vi "LidarLiteV3_I2C_Sample.vi"() -> ()   [LabVIEW 2019]
uses:
  <vilib>/ptbypt/NI_PtbyPt.lvlib
  <vilib>/Rock Robotics/SystemInterfaces/i2clib/i2c_bus.ctl
panel:
  out "Signal Stength":dbl format="%14.0f"
  in  "I2C Bus":T1
  in  "Average FIlter\nSamples":i32=5
  in  "Calibration\nOffset":dbl format="%#_13g"
  in  "Calibration \nGain":dbl=1.0 format="%#_13g"
  out "Lidar Distance Chart":cluster{dbl, "mean":dbl, dbl}(graph)
  out "Distance\nAverage FIlter\nFeet":dbl format="%19.3f"
  out "Distance\nFeet":dbl format="%19.3f"
  # "Read Lidar Lite V3 Using I2C Communications"
  # "Set these values before\nexecuting program"
  # "These values can be\nchanged while the \nprogram is running"
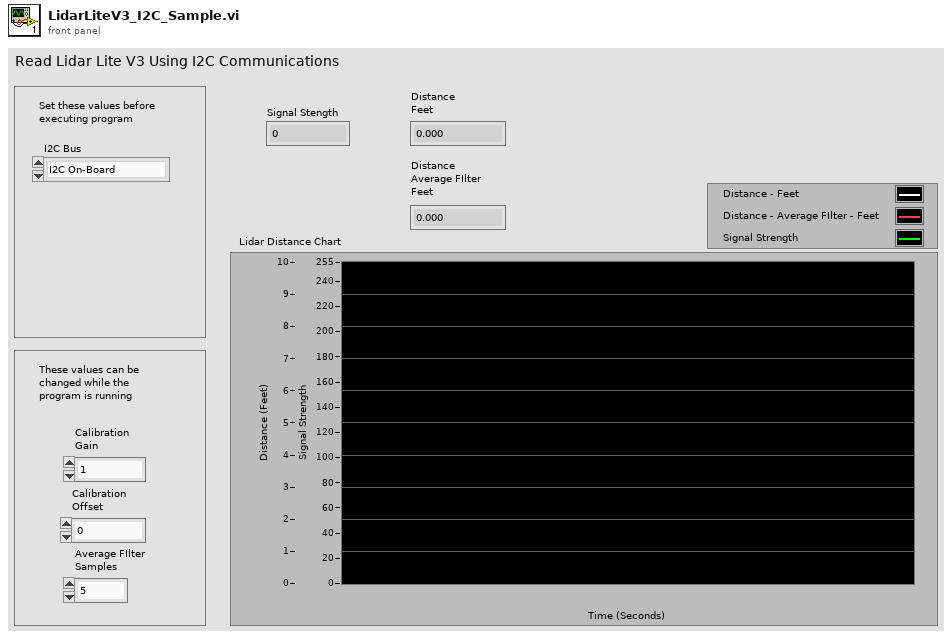
[diagram p1: front panel]
types:
  T1 = typedef "i2c_bus.ctl" = enum16{"I2C On-Board", "I2C MXP", "Invalid"}
  T2 = typedef "WPI_I2CDevRef.ctl" = cluster{"DevStatus":errorcluster, "Device Address":u8, "Handle":i32, "I2C Bus":T1}
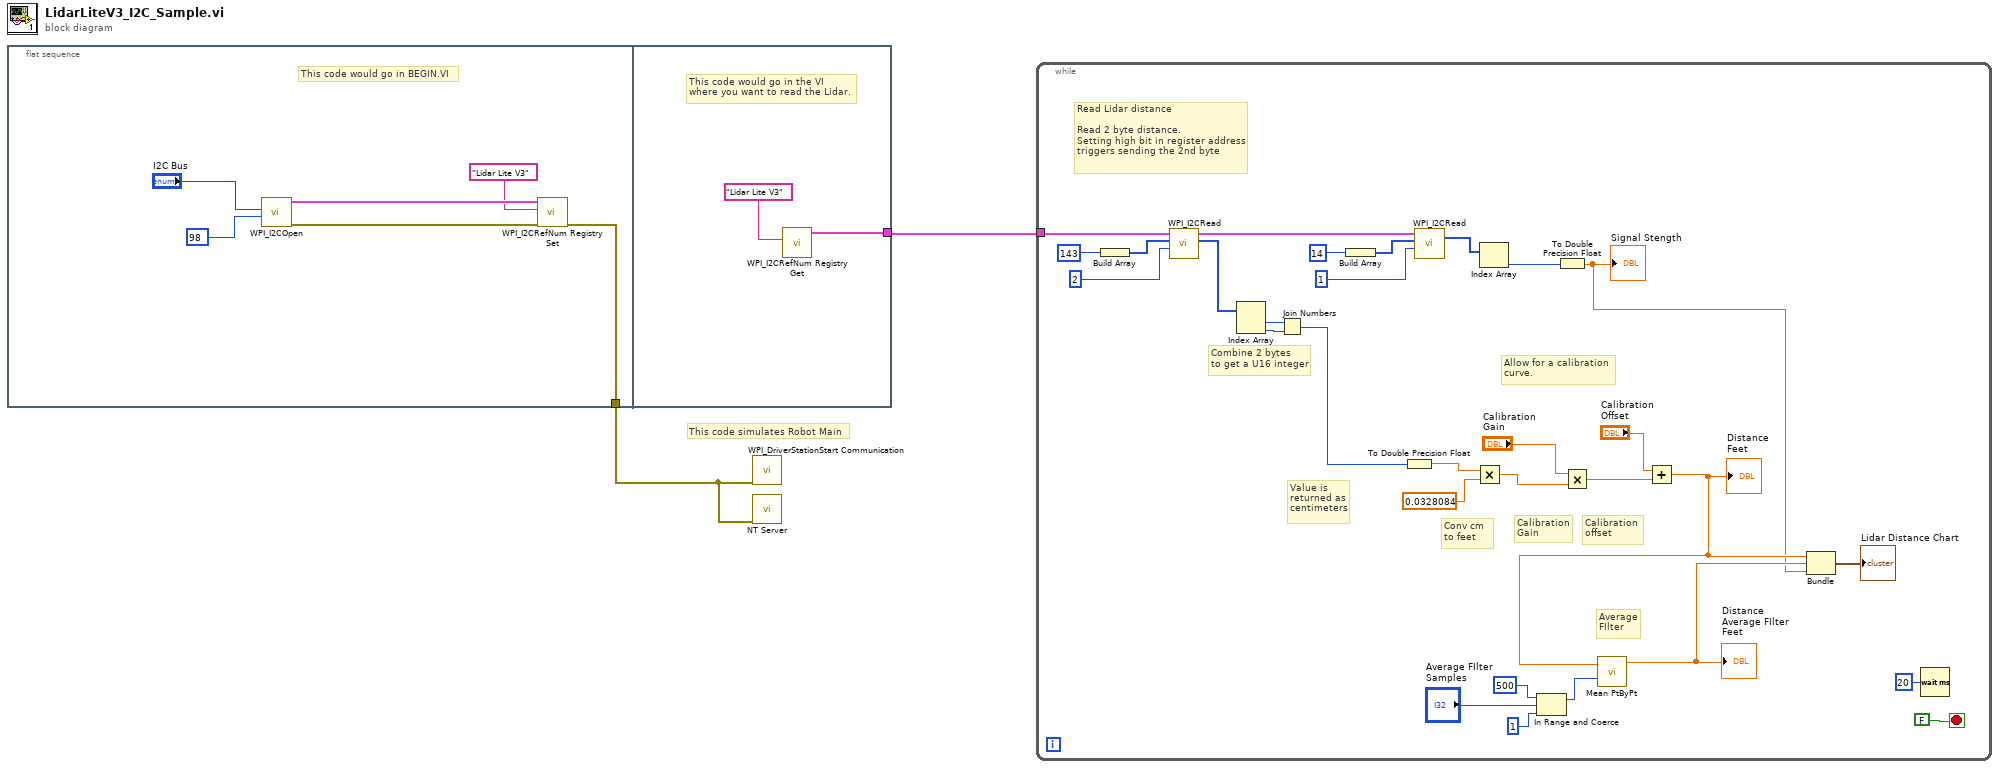
[diagram p0: block diagram]
diagram:
  # "This code simulates Robot Main"
  n1 = flat-sequence {
    tunnel: [w3] -> w1
    tunnel: [w9] -> w2
    frame #0 {
      # "This code would go in BEGIN.VI"
      n2 = call <vilib>:"WPI_I2COpen.vi"("Device Address"=u8 98, "I2C Bus"="I2C Bus") -> ("error out"=w6:errorcluster, "I2CDevRef"=w7:T2)  [unwired: 8 in]
      n3 = call <vilib>:"WPI_I2CRefNum Registry Set.vi"("error in (no error)"=w6, "refnum name"="Lidar Lite V3", "I2CDevRef"=w7) -> ("error out"=w3:errorcluster)  [unwired: 7 in, 1 out]
    }
    frame #1 {
      # "This code would go in the VI\nwhere you want to read the Lidar."
      n4 = call <vilib>:"WPI_I2CRefNum Registry Get.vi"("refnum name"="Lidar Lite V3") -> ("I2CDevRef"=w9:T2)  [unwired: 9 in, 1 out]
    }
  }
  n5 = call <vilib>:"WPI_DriverStationStart Communication.vi"("error in (no error)"=w1) -> ()  [unwired: 11 in]
  n6 = call <vilib>:"NT Server.vi"("error in (no error)"=w1) -> ()  [unwired: 11 in]
  n7 = while {
    tunnel: w2 -> [w26]
    stop <- FALSE stop-if-true
    # "Value is\nreturned as\ncentimeters"
    # "Combine 2 bytes\nto get a U16 integer"
    # "Average\nFIlter"
    # "Allow for a calibration\ncurve."
    # "Read Lidar distance\n\nRead 2 byte distance.\nSetting high bit in register address\ntriggers sending the 2nd byte"
    # "Calibration\nGain"
    # "Conv cm \nto feet"
    # "Calibration \noffset"
    n8 = Build Array(u8 143 ("Device Address")) -> (w24:u8[])
    n9 = call <vilib>:"WPI_I2CRead.vi"("I2CBytesToRead"=u8 2, "I2CRegister"=w24, "I2CDevRef"=w26) -> ("Data Out"=w22:u8[], "I2CDevRef"=w14:T2)  [unwired: 6 in, 1 out]
    n10 = Index Array(array=w22) -> (element #1=w20:u8, element #2=w21:u8)  [unwired: 2 in]
    n11 = Join Numbers(hi=w20, lo=w21) -> ((hi.lo)=w18:u16)
    n12 = Build Array(u8 14 ("Device Address")) -> (w16:u8[])
    n13 = To Double Precision Float(number=w18) -> (double precision float=w19:dbl)
    n14 = call <vilib>:"WPI_I2CRead.vi"("I2CBytesToRead"=u8 1, "I2CRegister"=w16, "I2CDevRef"=w14) -> ("Data Out"=w13:u8[])  [unwired: 6 in, 2 out]
    n15 = Multiply(x=w19, y=0.0328084) -> (x*y=w34:dbl)
    n16 = Index Array(array=w13) -> (element=w12:u8)  [unwired: 1 in]
    n17 = In Range and Coerce(upper limit=500, x="Average FIlter\nSamples", lower limit=1) -> (coerced(x)=w27:i32)  [unwired: 1 out]
    n18 = To Double Precision Float(number=w12) -> (double precision float=w11:dbl)
    "Signal Stength" <- w11
    n19 = Multiply(x="Calibration \nGain", y=w34) -> (x*y=w32:dbl)
    n20 = Add(x="Calibration\nOffset", y=w32) -> (x+y=w36:dbl)
    "Distance\nFeet" <- w36
    n21 = call <vilib>:"Mean PtByPt.vi"("x"=w36, "sample length"=w27) -> ("mean"=w35:dbl)  [unwired: 2 in, 1 out]
    "Distance\nAverage FIlter\nFeet" <- w35
    n22 = Bundle(w36, "mean"=w35, w11) -> (→"Lidar Distance Chart":cluster{dbl, "mean":dbl, dbl})  [unwired: 1 in]
    n23 = Wait (ms)(milliseconds to wait=u32 20) -> ()  [unwired: 1 out]
  }
